vi "Open Stimulus Profile Session.vi"(7 "Description":string, 8 "error in (no error)":errorcluster, 9 "Gateway IP Address (\"\": localhost)":string, 10 "Session Name":string, 11 "Sequence Calls":T2[](array[typedef])) -> (0 "error out":errorcluster, 3 "Session Ref":T1)   [LabVIEW 2020, in "NI_VS Sequence Execution Interface.lvlib"]
doc: "Connects to the VeriStand Gateway and creates a session with a name you specify."
uses:
  <vilib>/NI VeriStand/Execution/SequenceExecutionInterface/NI_VS Sequence Execution Interface.lvlib
  <vilib>/NI VeriStand/Execution/SequenceExecutionInterface/Sequence Call Ref.ctl
  NationalInstruments.VeriStand.ClientAPI
  <vilib>/NI VeriStand/Execution/SequenceExecutionInterface/Stimulus Profile Session Ref.ctl
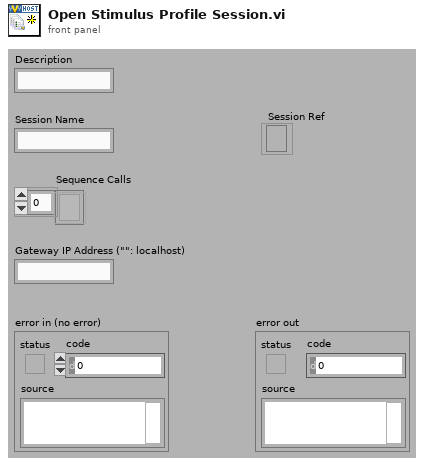
[diagram p1: front panel]
types:
  T1 = typedef "NI_VS Sequence Execution Interface.lvlib/Stimulus Profile Session Ref.ctl" = refnum<k24>
  T2 = typedef "NI_VS Sequence Execution Interface.lvlib/Sequence Call Ref.ctl" = refnum<k24>
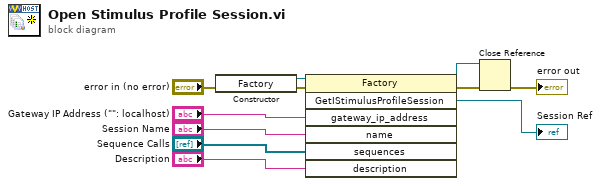
[diagram p0: block diagram]
diagram:
  n1 = constructor class="Factory"(error in="error in (no error)") -> (reference out=w10:refnum<k24>, error out=w11:errorcluster)  [unwired: 2 in, 1 out]
  n2 = invoke class="Factory" method="GetIStimulusProfileSession"(reference=w10, error in=w11, "gateway_ip_address"="Gateway IP Address (\"\": localhost)", "name"="Session Name", "sequences"="Sequence Calls", "description"="Description") -> (reference out=w2:refnum<k24>, error out=w3:errorcluster, "GetIStimulusProfileSession"=→"Session Ref":refnum<k24>)  [unwired: 1 in, 4 out]
  n3 = Close Reference(reference=w2, error in (no error)=w3) -> (error out=→"error out":errorcluster)
